vi "Convert Variant Parameters to FEDef.vi"(9 "error in":errorcluster, 10 "Variant Parameter Array":variant[](array[variant])) -> (1 "error out":errorcluster, 2 "FE_DEF":T1)   [LabVIEW 2011]
uses:
  Front End Definition.ctl
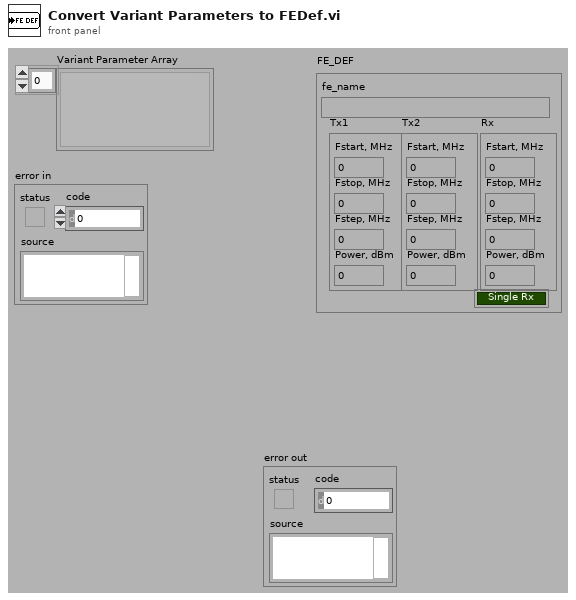
[diagram p1: front panel]
types:
  T1 = typedef "Front End Definition.ctl" = cluster{"fe_name":string, "Tx1":cluster{"Fstart, MHz":dbl, "Fstop, MHz":dbl, "Fstep, MHz":dbl, "Power, dBm":dbl}, "Tx2":cluster{"Fstart, MHz":dbl, "Fstop, MHz":dbl, "Fstep, MHz":dbl, "Power, dBm":dbl}, "Rx":cluster{"Fstart, MHz":dbl, "Fstop, MHz":dbl, "Fstep, MHz":dbl, "Power, dBm":dbl}, "BothSides":bool}
  T2 = cluster{"Fstart, MHz":dbl, "Fstop, MHz":dbl, "Fstep, MHz":dbl, "Power, dBm":dbl}
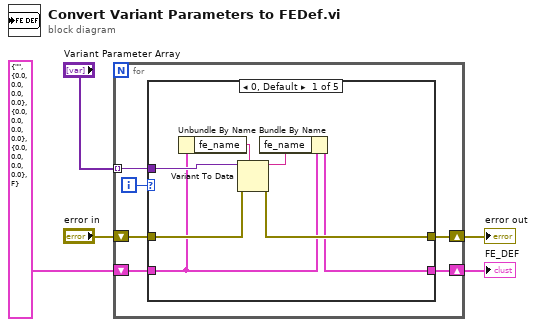
[diagram p0: block diagram]
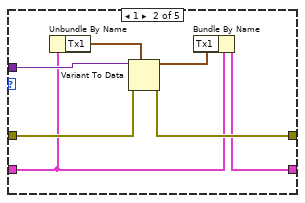
[diagram p2: hidden frame]
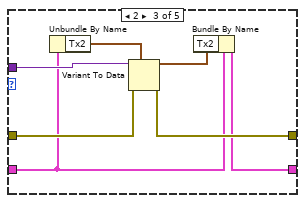
[diagram p3: hidden frame]
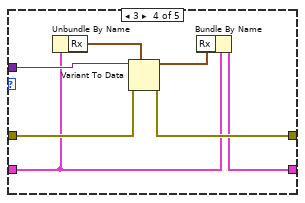
[diagram p4: hidden frame]
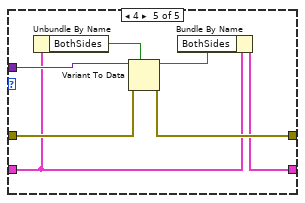
[diagram p5: hidden frame]
diagram:
  n1 = for {
    shift-right: [w10] -> w4
    shift-left: "error in" -> [w11]
    shift-right: [w7] -> w1
    shift-left: T1 {"fe_name"="", "Tx1"={"Fstart, MHz"=0.0, "Fstop, MHz"=0.0, "Fstep, MHz"=0.0, "Power, dBm"=0.0}, "Tx2"={"Fstart, MHz"=0.0, "Fstop, MHz"=0.0, "Fstep, MHz"=0.0, "Power, dBm"=0.0}, "Rx"={"Fstart, MHz"=0.0, "Fstop, MHz"=0.0, "Fstep, MHz"=0.0, "Power, dBm"=0.0}, "BothSides"=FALSE} ("FE_DEF") -> [w8]
    tunnel: "Variant Parameter Array" -> [w9] mode=indexing
    i -> [w6]
    n2 = case shown="0, Default" w6 {
      tunnel: w11 -> [w18 w25 w32 w39 w46]
      tunnel: [w17 w24 w31 w38 w45] -> w10
      tunnel: w9 -> [w16 w23 w30 w37 w44]
      tunnel: w8 -> [w13 w20 w27 w34 w41]
      tunnel: [w12 w19 w26 w33 w40] -> w7
      frame 0, Default {
        n3 = Unbundle By Name(w13) -> ("fe_name"=w15:string)
        n4 = Variant To Data(error in=w18, type=w15, Variant=w16) -> (data=w14:string, error out=w17:errorcluster)
        n5 = Bundle By Name(cluster=w13, "fe_name"=w14) -> (w12:T1)
      }
      frame 1 {
        n6 = Unbundle By Name(w20) -> ("Tx1"=w22:T2)
        n7 = Variant To Data(error in=w25, type=w22, Variant=w23) -> (data=w21:T2, error out=w24:errorcluster)
        n8 = Bundle By Name(cluster=w20, "Tx1"=w21) -> (w19:T1)
      }
      frame 2 {
        n9 = Unbundle By Name(w27) -> ("Tx2"=w29:T2)
        n10 = Variant To Data(error in=w32, type=w29, Variant=w30) -> (data=w28:T2, error out=w31:errorcluster)
        n11 = Bundle By Name(cluster=w27, "Tx2"=w28) -> (w26:T1)
      }
      frame 3 {
        n12 = Unbundle By Name(w34) -> ("Rx"=w36:T2)
        n13 = Variant To Data(error in=w39, type=w36, Variant=w37) -> (data=w35:T2, error out=w38:errorcluster)
        n14 = Bundle By Name(cluster=w34, "Rx"=w35) -> (w33:T1)
      }
      frame 4 {
        n15 = Unbundle By Name(w41) -> ("BothSides"=w43:bool)
        n16 = Variant To Data(error in=w46, type=w43, Variant=w44) -> (data=w42:bool, error out=w45:errorcluster)
        n17 = Bundle By Name(cluster=w41, "BothSides"=w42) -> (w40:T1)
      }
    }
  }
  "error out" <- w4
  "FE_DEF" <- w1
